vi "Merge Configuration.vi"(8 "error in (no error)":errorcluster, 10 "Configuration to Merge":refnum<class "Column Configuration.lvclass">, 11 "Column Configuration in":refnum<class "Column Configuration.lvclass">) -> (0 "error out":errorcluster, 3 "Column Configuration out":refnum<class "Column Configuration.lvclass">)   [LabVIEW 2020, in "Column Interfaces.lvlib" / "Column Configuration.lvclass"]
uses:
  Column Configuration.lvclass
  Column Configuration.lvclass/Column Configuration.ctl
  Database Libraries/Database Interfaces/Database Interface Class/Database Interface.lvclass
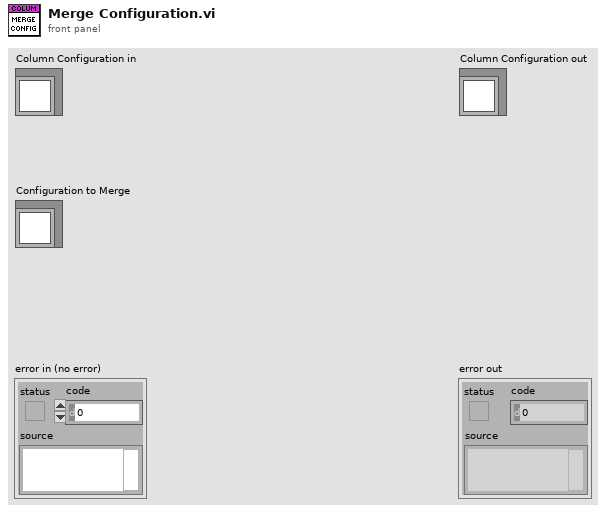
[diagram p1: front panel]
types:
  T1 = typedef "Database Interfaces.lvlib/Database data type.ctl" = enum16{"Undefined", "String", "Long (I32)", "Single (SGL)", "Double (DBL)", "Date/Time", "Binary"}
  T2 = typedef "Column Interfaces.lvlib/FK Info.ctl" = cluster{"PK Table":string, "PK Column":string, "PK Display Column":string}
  T3 = typedef "Database Interfaces.lvlib/Primary Key Info.ctl" = cluster{"Primary Key Column":string, "Display Column":string}
  T4 = cluster{"Table Name":string, "Column Name":string, "Column Type":T1, "Database":refnum<class "Database Interface.lvclass">, "FK Info":T2, "Primary Key":T3}
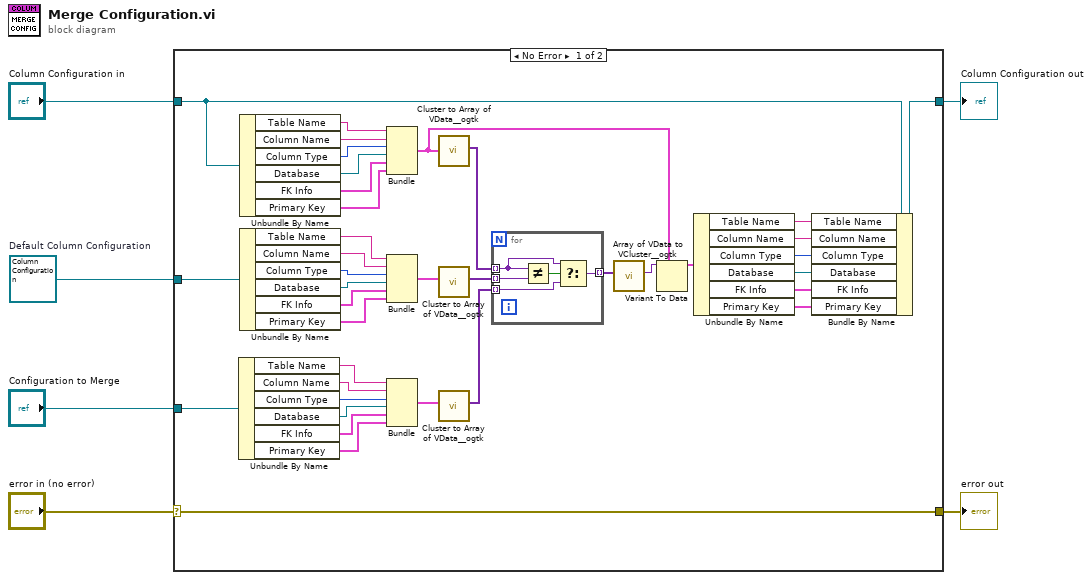
[diagram p0: block diagram]
diagram:
  w1 = refnum<class "Column Configuration.lvclass"> refnum  # Default Column Configuration
  n1 = case shown="No Error" "error in (no error)" {
    selector: "error in (no error)" -> [w44 w51]
    tunnel: [w44 w51] -> w5
    tunnel: [w13 w50] -> w3
    tunnel: "Column Configuration in" -> [w14 w50]
    tunnel: "Configuration to Merge" -> [w42 _]
    tunnel: w1 -> [w43 _]
    frame No Error {
      n2 = Unbundle By Name(w42) -> ("Table Name"=w29:string, "Column Name"=w28:string, "Column Type"=w27:T1, "Database"=w26:refnum<class "Database Interface.lvclass">, "FK Info"=w25:T2, "Primary Key"=w24:T3)
      n3 = Unbundle By Name(w14) -> ("Table Name"=w41:string, "Column Name"=w40:string, "Column Type"=w39:T1, "Database"=w38:refnum<class "Database Interface.lvclass">, "FK Info"=w37:T2, "Primary Key"=w36:T3)
      n4 = Unbundle By Name(w43) -> ("Table Name"=w35:string, "Column Name"=w34:string, "Column Type"=w33:T1, "Database"=w32:refnum<class "Database Interface.lvclass">, "FK Info"=w31:T2, "Primary Key"=w30:T3)
      n5 = Bundle("Table Name"=w41, "Column Name"=w40, "Column Type"=w39, "Database"=w38, "FK Info"=w37, "Primary Key"=w36) -> (w16:T4)  [unwired: 1 in]
      n6 = Bundle("Table Name"=w35, "Column Name"=w34, "Column Type"=w33, "Database"=w32, "FK Info"=w31, "Primary Key"=w30) -> (w23:T4)  [unwired: 1 in]
      n7 = Bundle("Table Name"=w29, "Column Name"=w28, "Column Type"=w27, "Database"=w26, "FK Info"=w25, "Primary Key"=w24) -> (w22:T4)  [unwired: 1 in]
      n8 = call <userlib>:"Cluster to Array of VData__ogtk.vi"("Cluster"=w16) -> ("Array of VData"=w21:variant[])  [unwired: 9 in, 1 out]
      n9 = call <userlib>:"Cluster to Array of VData__ogtk.vi"("Cluster"=w23) -> ("Array of VData"=w20:variant[])  [unwired: 9 in, 1 out]
      n10 = call <userlib>:"Cluster to Array of VData__ogtk.vi"("Cluster"=w22) -> ("Array of VData"=w19:variant[])  [unwired: 9 in, 1 out]
      n11 = for {
        tunnel: w21 -> [w46] mode=indexing
        tunnel: w20 -> [w49] mode=indexing
        tunnel: w19 -> [w48] mode=indexing
        tunnel: [w45] -> w18 mode=indexing
        n12 = Not Equal?(x=w46, y=w49) -> (x != y?=w47:bool)
        n13 = Select(t=w46, s=w47, f=w48) -> (s? t:f=w45:variant)
      }
      n14 = call <userlib>:"Array of VData to VCluster__ogtk.vi"("Array"=w18) -> ("VCluster"=w17:variant)  [unwired: 9 in, 1 out]
      n15 = Variant To Data(type=w16, Variant=w17) -> (data=w12:T4)  [unwired: 1 in, 1 out]
      n16 = Unbundle By Name(w12) -> ("Table Name"=w7:string, "Column Name"=w8:string, "Column Type"=w9:T1, "Database"=w10:refnum<class "Database Interface.lvclass">, "FK Info"=w11:T2, "Primary Key"=w15:T3)
      n17 = Bundle By Name(cluster=w14, "Table Name"=w7, "Column Name"=w8, "Column Type"=w9, "Database"=w10, "FK Info"=w11, "Primary Key"=w15) -> (w13:refnum<class "Column Configuration.lvclass">)
    }
    frame Error {
    }
  }
  "error out" <- w5
  "Column Configuration out" <- w3
